vi "Read LimitOverride.vi"(8 "error in (no error)":errorcluster, 11 "SignalWithAlarm in":refnum<class "SignalWithAlarm.lvclass">) -> (0 "error out":errorcluster, 2 "LimitOverride":refnum<user-event>, 3 "SignalWithAlarm out":refnum<class "SignalWithAlarm.lvclass">)   [LabVIEW 2016, in "SignalWithAlarm.lvclass"]
uses:
  SignalWithAlarm.lvclass
  SignalWithAlarm.lvclass/SignalWithAlarm.ctl
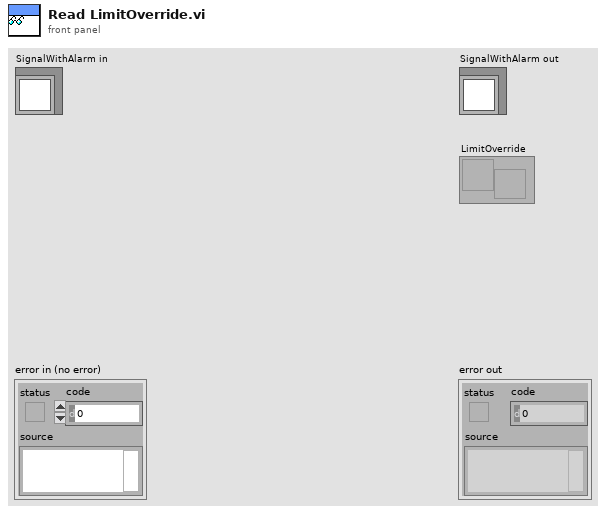
[diagram p1: front panel]
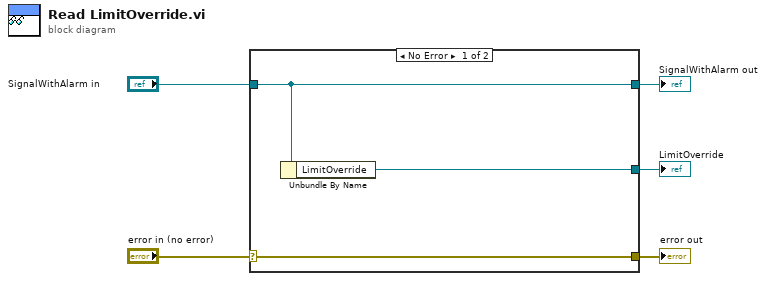
[diagram p0: block diagram]
diagram:
  n1 = case shown="No Error" "error in (no error)" {
    selector: "error in (no error)" -> [w8 w9]
    tunnel: [w8 w9] -> w4
    tunnel: [w7 w10] -> w2
    tunnel: "SignalWithAlarm in" -> [w7 w10]
    tunnel: [w6 _] -> w1
    frame No Error {
      n2 = Unbundle By Name(w7) -> ("LimitOverride"=w6:refnum<user-event>)
    }
    frame Error {
    }
  }
  "error out" <- w4
  "SignalWithAlarm out" <- w2
  "LimitOverride" <- w1
